vi "Apply Config.vi"(8 "ErrorIn":errorcluster, 10 "Name":string, 11 "TopModuleIn":refnum<class "LoggerAPI.lvclass">) -> (0 "ErrorOut":errorcluster, 3 "TopModuleOut":refnum<class "LoggerAPI.lvclass">)   [LabVIEW 2020, in "LoggerAPI.lvclass"]
uses:
  LoggerAPI.lvclass
  IConfig/IConfig.lvclass
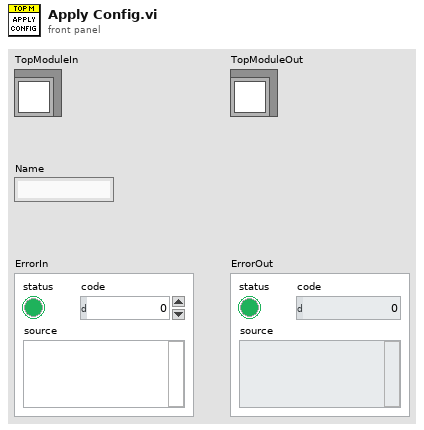
[diagram p1: front panel]
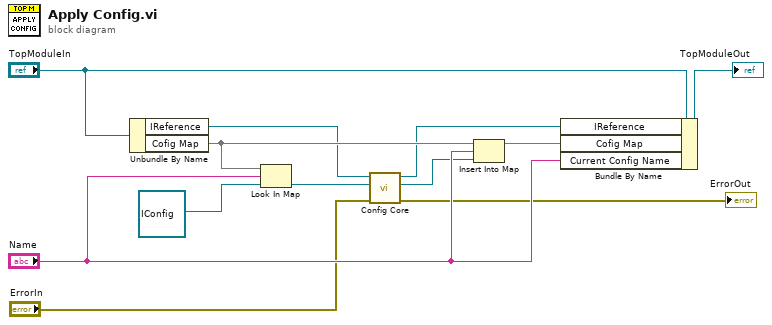
[diagram p0: block diagram]
diagram:
  n1 = Unbundle By Name("TopModuleIn") -> ("IReference"=w6:refnum<class "IRef.lvclass">, "Cofig Map"=w10:map{string, refnum<class "IConfig.lvclass">})
  n2 = Look In Map(map=w10, key="Name", default value=refnum<class "IConfig.lvclass"> refnum ("IConfig.lvclass")) -> (value=w5:refnum<class "IConfig.lvclass">)  [unwired: 1 out]
  n3 = call-dynamic "Config Core.vi"("Error In"="ErrorIn", "IConfig In"=w5, "Hardware In"=w6) -> ("Error Out"=→"ErrorOut":errorcluster, "IConfig Out"=w2:refnum<class "IConfig.lvclass">, "Hardware Out"=w1:refnum<class "IRef.lvclass">)  [unwired: 6 in]
  n4 = Insert Into Map(map in=w10, key="Name", value=w2) -> (map out=w9:map{string, refnum<class "IConfig.lvclass">})  [unwired: 2 out]
  n5 = Bundle By Name(cluster="TopModuleIn", "IReference"=w1, "Cofig Map"=w9, "Current Config Name"="Name") -> (→"TopModuleOut":refnum<class "LoggerAPI.lvclass">)
